vi "[SubVI]Matrix_Math.vi"(5 "Computed Features":dbl[](array[numeric]), 7 "NN Matrix":T2) -> (3 "Gait Phase":dbl)   [LabVIEW 2018]
uses:
  <vilib>/Analysis/Matrix/Datatypes/RealMatrix.ctl
  <vilib>/Analysis/Matrix/Numeric/Conversions/Array To Matrix - RA.vi
  <vilib>/Analysis/Matrix/Numeric/Multiply/Multiply - RM,RM.vi
  <vilib>/Analysis/Matrix/Numeric/Add/Add - RM,RM.vi
  <vilib>/Analysis/Matrix/NI_Matrix.lvlib
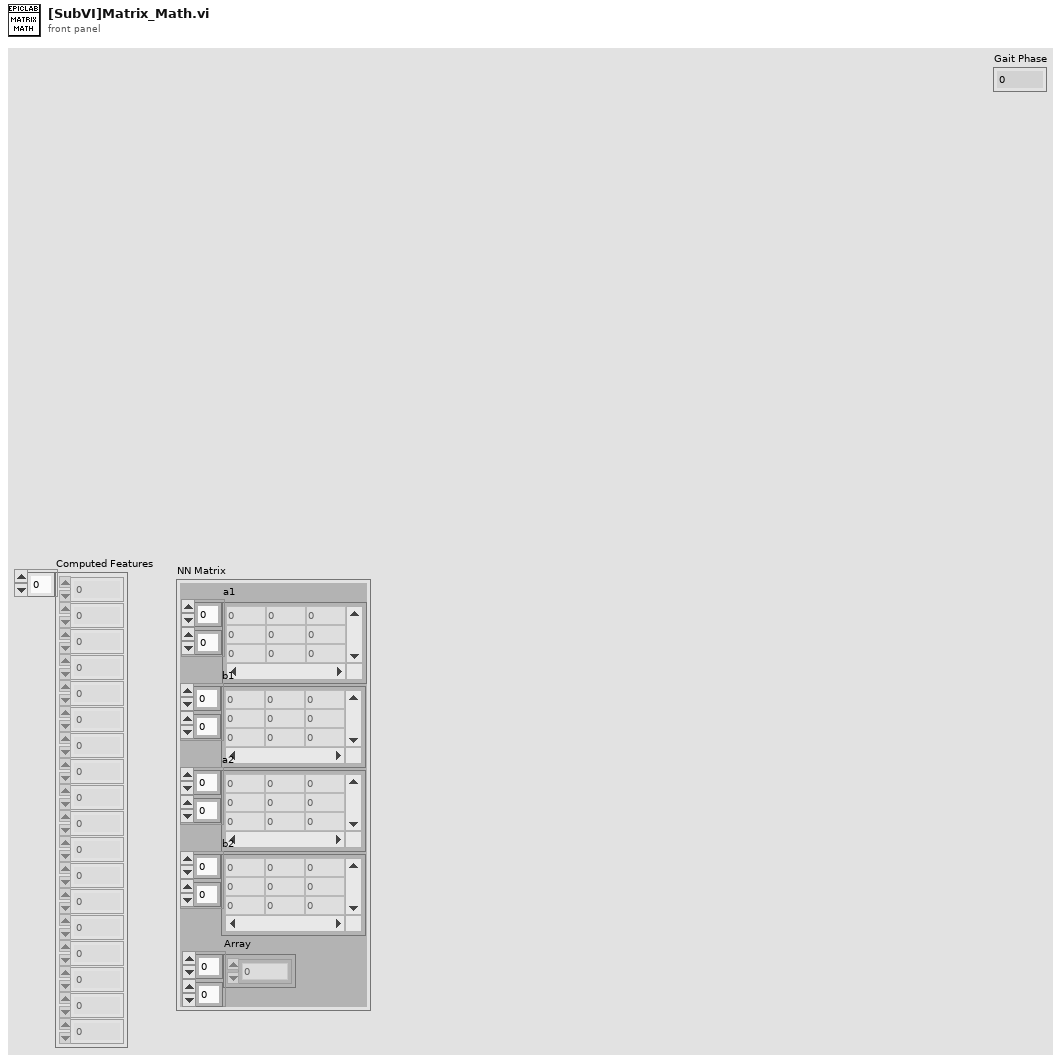
[diagram p1: front panel]
types:
  T1 = typedef "NI_Matrix.lvlib/RealMatrix.ctl" = dbl[][]
  T2 = cluster{"a1":T1, "b1":T1, "a2":T1, "b2":T1, "Array":dbl[][]}
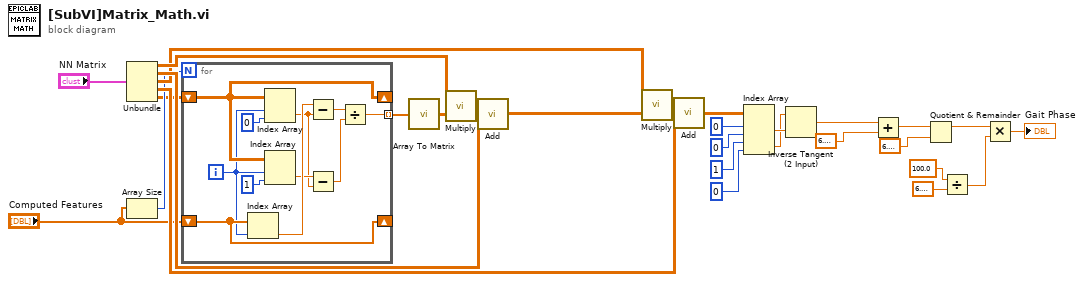
[diagram p0: block diagram]
diagram:
  n1 = Unbundle("NN Matrix") -> ("a1"=w24:T1, "b1"=w27:T1, "a2"=w22:T1, "b2"=w25:T1, "Array"=w8:dbl[][])
  n2 = Array Size(array="Computed Features") -> (size(s)=w9:i32)
  n3 = for {
    N: w9 -> [_]
    shift-right: [w38] -> _
    shift-left: w8 -> [w38]
    shift-right: [w37] -> _
    shift-left: "Computed Features" -> [w37]
    tunnel: [w30] -> w6 mode=indexing
    i -> [w36]
    n4 = Index Array(array=w37, index=w36) -> (element=w35:dbl)
    n5 = Index Array(array=w38, index (row)=w36, index (col)=0 ("disabled index (col)")) -> (element=w33:dbl)
    n6 = Index Array(array=w38, index (row)=w36, index (col)=1 ("disabled index (col)")) -> (element=w34:dbl)
    n7 = Subtract(x=w35, y=w33) -> (x-y=w32:dbl)
    n8 = Subtract(x=w34, y=w33) -> (x-y=w31:dbl)
    n9 = Divide(x=w32, y=w31) -> (x/y=w30:dbl)
  }
  n10 = call-poly <vilib>:"Array To Matrix.vi"("Real 1D Array"=w6) -> ("Real Matrix (Column Vector)"=w23:T1)
  n11 = call-poly <vilib>:"Multiply.vi"("Real Matrix B"=w23, "Real Matrix A"=w24) -> ("A * B"=w28:T1)
  n12 = call-poly <vilib>:"Add.vi"("Real Matrix B"=w27, "Real Matrix A"=w28) -> ("A + B"=w1:T1)
  n13 = call-poly <vilib>:"Multiply.vi"("Real Matrix B"=w1, "Real Matrix A"=w22) -> ("A * B"=w26:T1)
  n14 = call-poly <vilib>:"Add.vi"("Real Matrix B"=w25, "Real Matrix A"=w26) -> ("A + B"=w21:T1)
  n15 = Index Array(array=w21, index (row) #1=0 ("index (row)"), index (col) #1=0 ("index (col)"), index (row) #2=1 ("index (row)"), index (col) #2=0 ("index (col)")) -> (element #1=w16:dbl, element #2=w15:dbl)
  n16 = Inverse Tangent (2 Input)(1:w16, 2:w15) -> (0:w14:dbl)
  n17 = Add(x=w14, y=6.283185307179586) -> (x+y=w3:dbl)
  n18 = Quotient & Remainder(x=w3, y=6.283185307179586) -> (x-y*floor(x/y)=w2:dbl)  [unwired: 1 out]
  n19 = Divide(x=100.0, y=6.283185307179586) -> (x/y=w11:dbl)
  n20 = Multiply(x=w2, y=w11) -> (x*y=→"Gait Phase":dbl)
